vi "ArmController.vi"(7 "Force Value":i32, 9 "State":i32, 10 "Level":i32) -> (1 "Setpoint":i32)   [LabVIEW 2014]
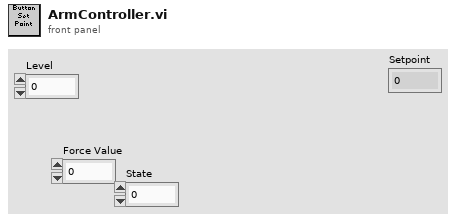
[diagram p1: front panel]
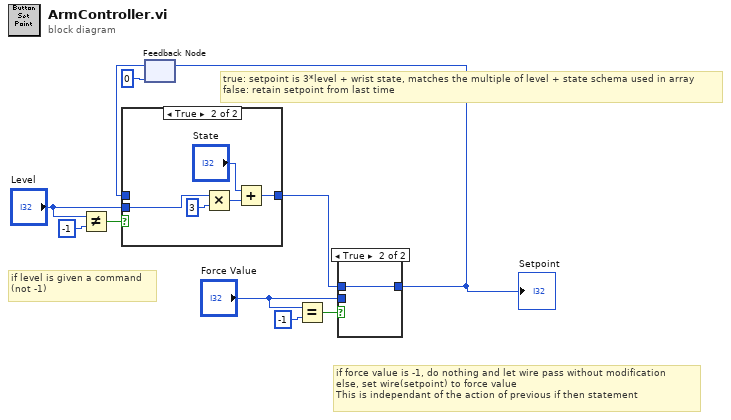
[diagram p0: block diagram]
diagram:
  # "if force value is -1, do nothing and let wire pass without modification\nelse, set wire(setpoint) to force value\nThis is independant of the action of previous if then statement"
  # "true: setpoint is 3*level + wrist state, matches the multiple of level + state schema used in array\nfalse: retain setpoint from last time"
  # "if level is given a command\n(not -1)"
  n1 = Not Equal?(x="Level", y=-1) -> (x != y?=w2:bool)
  n2 = feedback #1(0) -> (w5:i32)
  n3 = case shown="True" w2 {
    tunnel: "Level" -> [_ w13]
    tunnel: [w11 w12] -> w7
    tunnel: w5 -> [w11 _]
    frame False {
    }
    frame True {
      n4 = Multiply(x=w13, y=3) -> (x*y=w15:i32)
      n5 = Add(x="State", y=w15) -> (x+y=w12:i32)
    }
  }
  n6 = Equal?(x="Force Value", y=-1) -> (x = y?=w9:bool)
  n7 = case shown="True" w9 {
    tunnel: w7 -> [_ w18]
    tunnel: [w17 w18] -> w1
    tunnel: "Force Value" -> [w17 _]
    frame False {
    }
    frame True {
    }
  }
  "Setpoint" <- w1
  n8 = feedback-in #1(w1) -> ()
